vi "Dlg-New-Portfolio.vi"(7 "Config File Path":path, 8 "error in (no error)":errorcluster, 11 "Portfolio":refnum<class "Portfolio.lvclass">) -> (0 "error out":errorcluster, 2 "Canceled":bool, 3 "Portfolio out":refnum<class "Portfolio.lvclass">)   [LabVIEW 2012, in "Portfolio.lvclass"]
uses:
  Portfolio.lvclass
  Portfolio.lvclass/Portfolio.ctl
panel:
  out "path":path caption="chemin sélectionné"
  in  "Save":bool
  in  "Date de création":timestamp format="%<%X\n%x>T"
  in  "Nom du portefeuille":string
  in  "Cancel Button":bool
  in  "OK Button":bool
  in  "Help":bool
  # "Nouveau Portefeuille"
  # "Créer un nouveau Portefeuille"
  # "Portefeuille"
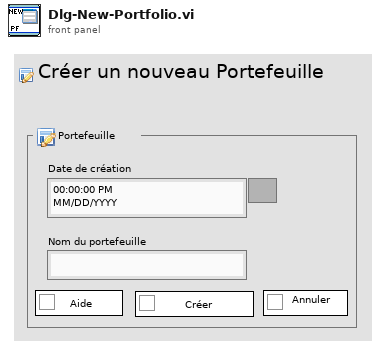
[diagram p1: front panel]
types:
  T1 = typedef "Portfolio Parameters.ctl" = cluster{"Date":timestamp, "Name":string, "Cash":dbl}
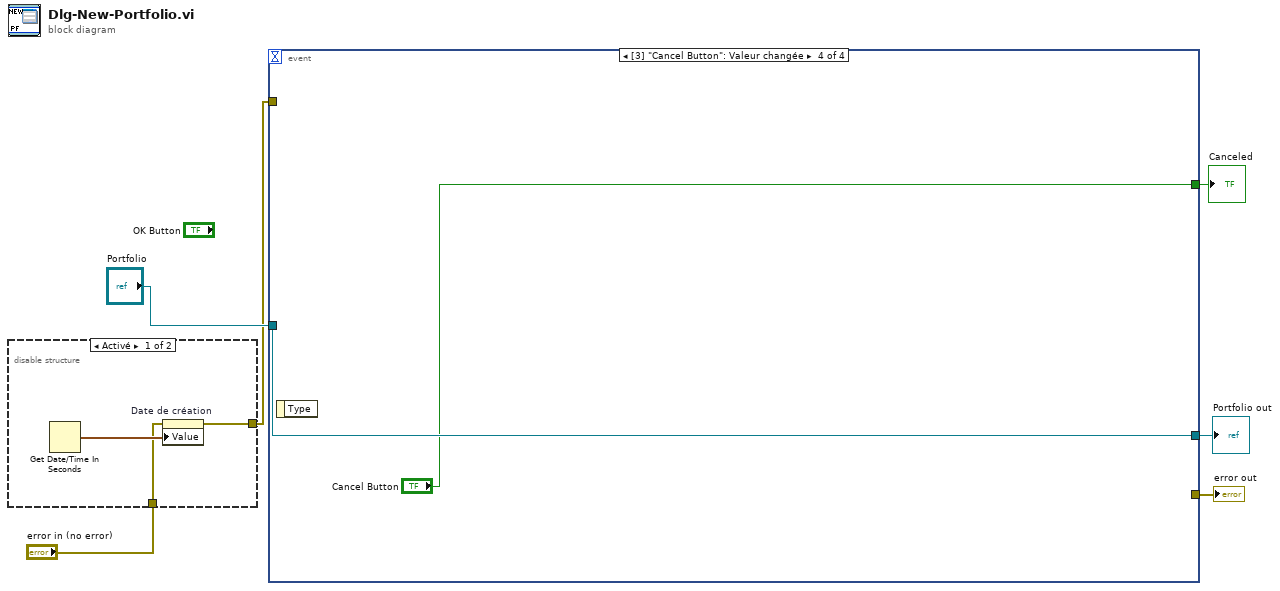
[diagram p0: block diagram]
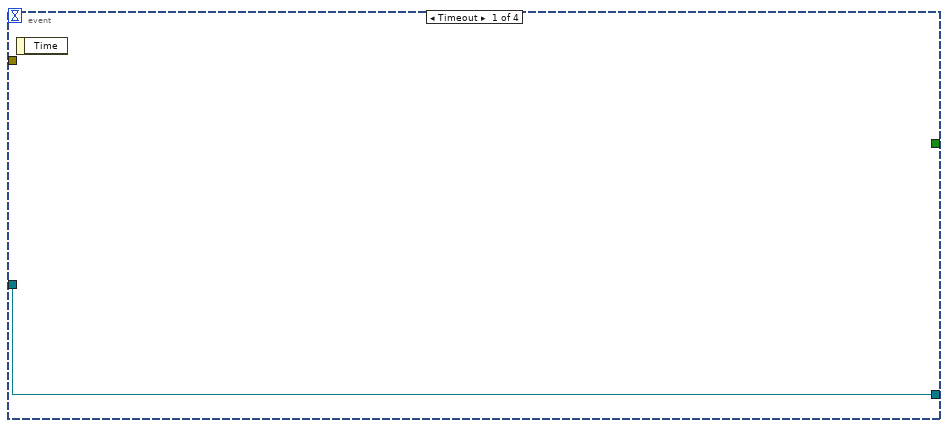
[diagram p3: hidden frame]
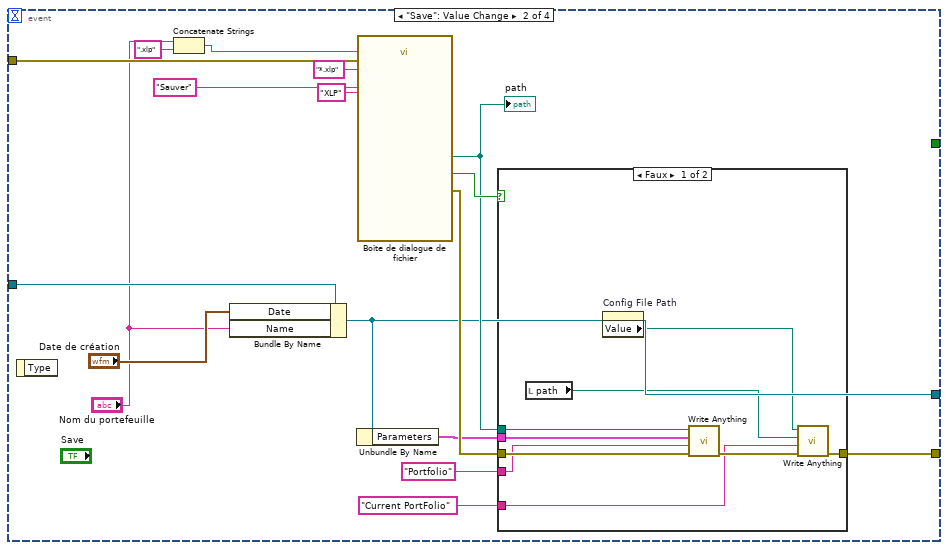
[diagram p4: hidden frame]
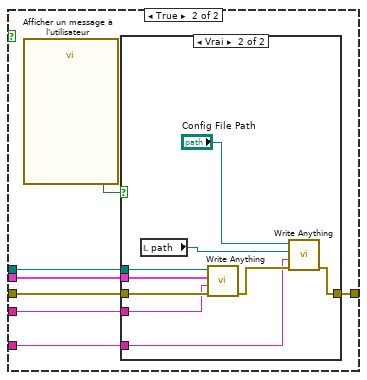
[diagram p5: hidden frame]
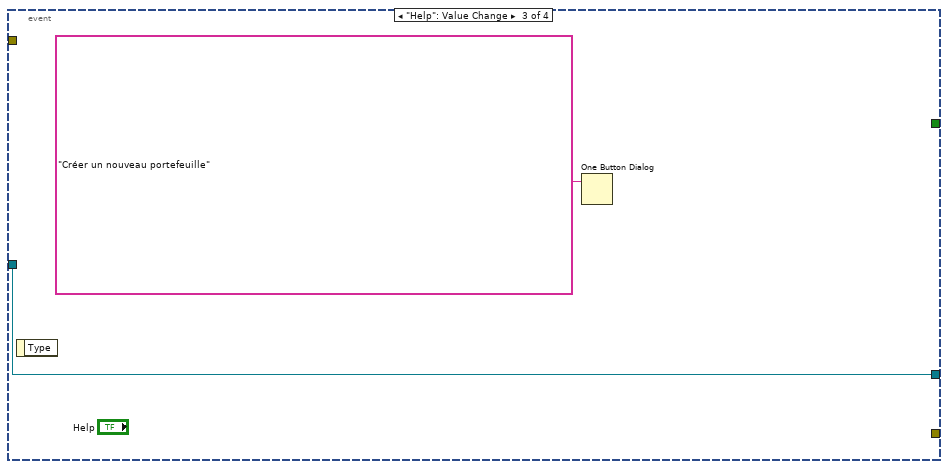
[diagram p7: hidden frame]
diagram:
  n1 = disable-structure shown="Activé" {
    disable-tunnel: [w8 _] -> w4
    disable-tunnel: "error in (no error)" -> [w7 _]
    frame Enabled {
      n2 = Get Date/Time In Seconds() -> (seconds since 1Jan1904=w9:timestamp)
      n3 = property on="Date de création" class="TempsAbs (strict)"(error in=w7, "Value"=w9) -> (error out=w8:errorcluster)  [unwired: 1 in, 1 out]
    }
    frame Disabled {
    }
  }
  n4 = event shown="[3] \"Cancel Button\": Valeur changée" {
    selector: _ -> [_ _ _ _]
    dyn-events: _ -> [_ _ _ _]
    timeout: _ -> [_ _ _ _]
    tunnel: [w10 w13 w55 w57] -> w6
    tunnel: "Portfolio" -> [w10 w27 w55 w57]
    tunnel: w4 -> [_ w24 _ _]
    tunnel: [_ w26 _ _] -> w2
    tunnel: [_ _ _ "Cancel Button"] -> w1
    event Timeout {
      n5 = event-data() -> ()  [unwired: 1 in, 1 out]
    }
    event "Save": Value Change {
      n6 = event-data() -> ()  [unwired: 1 in, 1 out]
      n7 = Concatenate Strings("Nom du portefeuille", ".xlp" ("chaîne")) -> (w18:string)
      n8 = Bundle By Name(cluster=w27, "Date"="Date de création", "Name"="Nom du portefeuille") -> (w13:refnum<class "Portfolio.lvclass">)
      n9 = Unbundle By Name(w13) -> ("Parameters"=w12:T1)
      n10 = call "Boîte de dialogue de fichier"("button label"="Sauver", "default name"=w18, "error in"=w24, "pattern (all files)"="*.xlp", "pattern label"="XLP") -> ("selected path"=w15:path, "exists"=w16:bool, "error out"=w25:errorcluster)  [unwired: 7 in, 1 out]
      "path" <- w15
      n11 = case shown="Faux" w16 {
        tunnel: [w32 w41] -> w26
        tunnel: w15 -> [w30 w42]
        tunnel: w25 -> [w36 w40]
        tunnel: "Portfolio" ("button label") -> [w35 w39]
        tunnel: w12 -> [w31 w38]
        tunnel: "Current PortFolio" ("button label") -> [w29 w37]
        frame False {
          n12 = local read "path"() -> (w28:path)
          n13 = property on="Config File Path" class="Chm"() -> ("Value"=w34:path)  [unwired: 2 in, 2 out]
          n14 = call "Write Anything.vi"("Error In"=w36, "Section Name (Name of \"Anything\")"=w35, "Anything"=w31, "Path (dialog)"=w30) -> ("Error Out"=w33:errorcluster)  [unwired: 7 in]
          n15 = call "Write Anything.vi"("Error In"=w33, "Section Name (Name of \"Anything\")"=w29, "Anything"=w28, "Path (dialog)"=w34) -> ("Error Out"=w32:errorcluster)  [unwired: 7 in]
        }
        frame True {
          n16 = call "Afficher un message à l'utilisateur"() -> ("OK"=w43:bool)  [unwired: 10 in, 1 out]
          n17 = case shown="Vrai" w43 {
            tunnel: w42 -> [_ w47]
            tunnel: [w44 w50] -> w41
            tunnel: w40 -> [w44 w53]
            tunnel: w39 -> [_ w49]
            tunnel: w38 -> [_ w48]
            tunnel: w37 -> [_ w46]
            frame False {
            }
            frame True {
              n18 = local read "path"() -> (w45:path)
              n19 = call "Write Anything.vi"("Error In"=w53, "Section Name (Name of \"Anything\")"=w49, "Anything"=w48, "Path (dialog)"=w47) -> ("Error Out"=w51:errorcluster)  [unwired: 7 in]
              n20 = call "Write Anything.vi"("Error In"=w51, "Section Name (Name of \"Anything\")"=w46, "Anything"=w45, "Path (dialog)"="Config File Path") -> ("Error Out"=w50:errorcluster)  [unwired: 7 in]
            }
          }
        }
      }
    }
    event "Help": Value Change {
      n21 = event-data() -> ()  [unwired: 1 in, 1 out]
      n22 = One Button Dialog(message="Créer un nouveau portefeuille") -> ()  [unwired: 1 in, 1 out]
    }
    event "Cancel Button": Value Change {
      n23 = event-data() -> ()  [unwired: 1 in, 1 out]
    }
  }
  "error out" <- w2
  "Portfolio out" <- w6
  "Canceled" <- w1
